vi "Synapse CCD (No Objects).vi"(8 "error in (no error)":errorcluster, 10 "Mono Unique ID":string="Mono1", 11 "Unique ID":string="CCD1") -> (0 "error out":errorcluster, 3 "Synapse CCD out":T1={"JYCCDLib.IJYCCDReqd"=refnum, "JYMONOLib.IJYMonoReqd"=refnum, "Integration time"=0.01, "ADC"=0, "GAIN"=0, "areas :"=[[1, 1, 1, 1024, 256, 1, 256]], "Most Recent Data Object"=refnum, "Mono Properties"={"Grating"=0, "Center Wavelength"=0.0, "Entrance Slit"=0.0, "Exit Slit"=0.0}, "Coverage"={"Max"=0.0, "Min"=0.0}, "Multi-Acquisitions"={"Dark Subtract?"=FALSE, "Averaging?"=FALSE, "Cosmic Ray Removal?"=FALSE, "# to Average"=0, "Time Between Acq."=0, "Acquisitions Control Array"=[TRUE], "Raw Data"=[], "Processed Data"=[], "Array of Wavelengths"=[]}, "Channel Names"=["Wavelength", "Signal"], "Channel Units"=["nm", "counts"]} {"ADC" items=["   20 kHz", "1 MHz", "1 MHz Ultra"]; "GAIN" items=["High Light", "Best Dynamic", "High Sensitivity"]; "Mono Properties"."Grating" items=["1200 lines/mm - 500 nm Blaze", "1200 lines/mm - 750 nm Blaze", "600 lines/mm - 1000 nm Blaze"]})   [LabVIEW 2015]
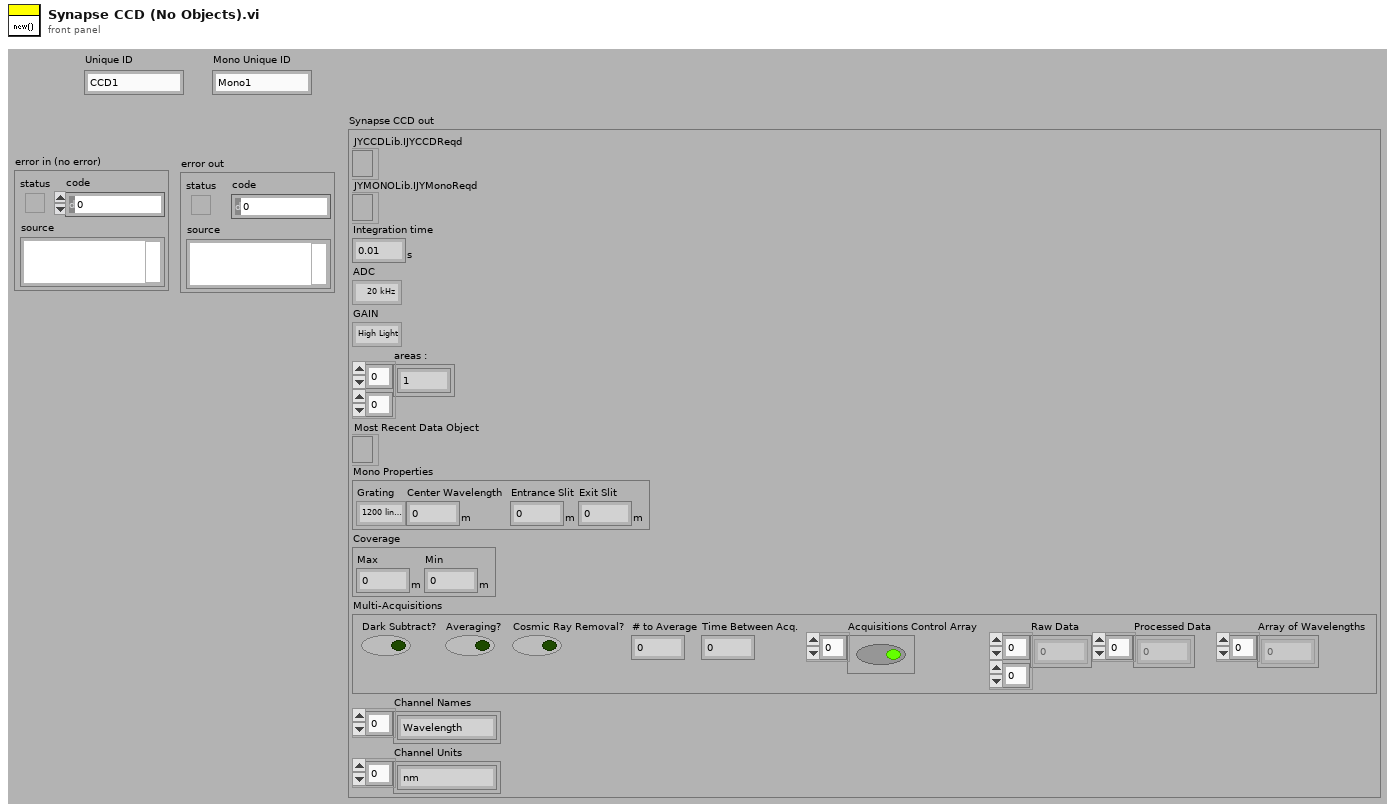
[diagram p1: front panel]
types:
  T1 = cluster{"JYCCDLib.IJYCCDReqd":refnum<k7>, "JYMONOLib.IJYMonoReqd":refnum<k7>, "Integration time":dbl[unit], "ADC":u16, "GAIN":u16, "areas :":i32[][], "Most Recent Data Object":refnum<k7>, "Mono Properties":cluster{"Grating":u16, "Center Wavelength":dbl[unit], "Entrance Slit":dbl[unit], "Exit Slit":dbl[unit]}, "Coverage":cluster{"Max":dbl[unit], "Min":dbl[unit]}, "Multi-Acquisitions":cluster{"Dark Subtract?":bool, "Averaging?":bool, "Cosmic Ray Removal?":bool, "# to Average":u32, "Time Between Acq.":u32, "Acquisitions Control Array":bool[], "Raw Data":i32[][], "Processed Data":dbl[], "Array of Wavelengths":dbl[]}, "Channel Names":string[], "Channel Units":string[]}
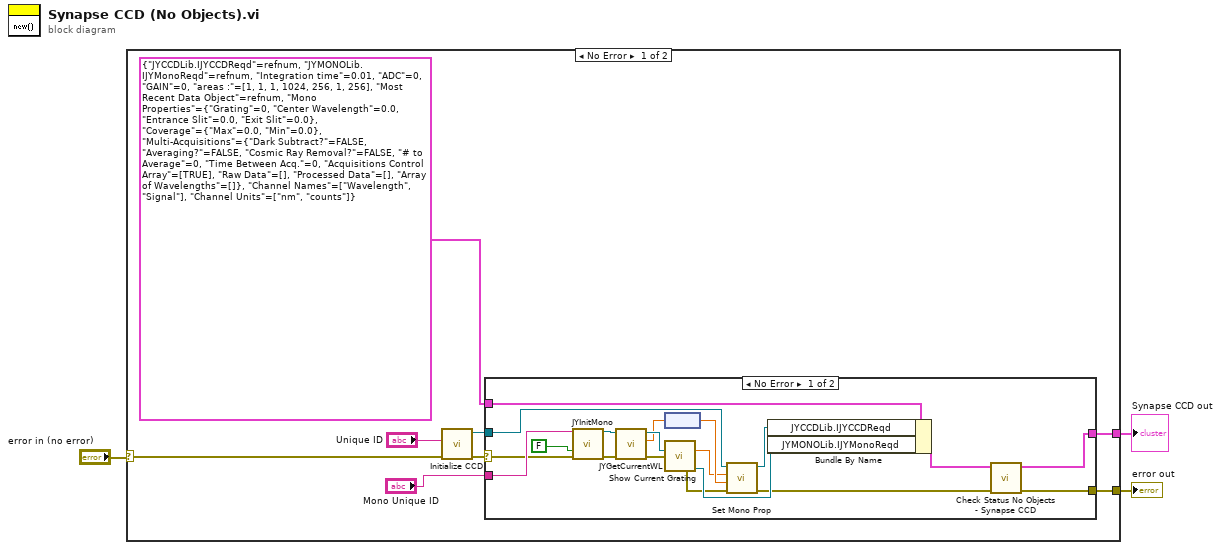
[diagram p0: block diagram]
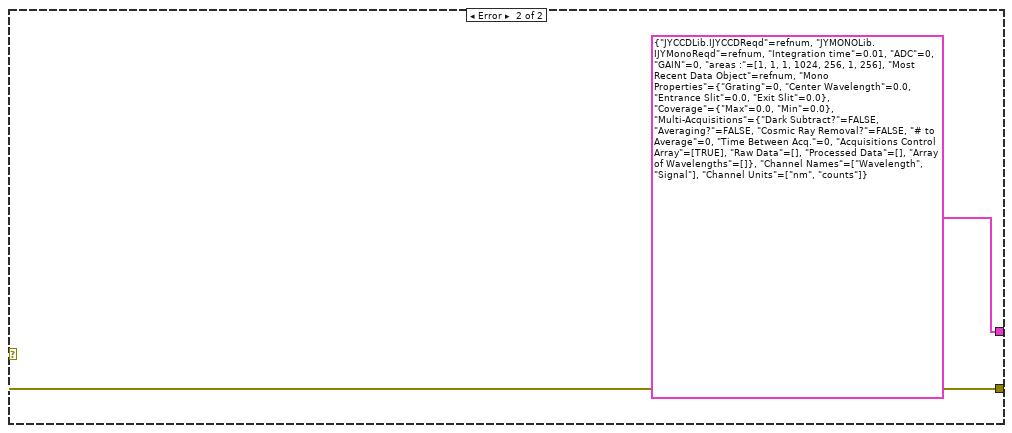
[diagram p3: hidden frame]
diagram:
  n1 = case shown="No Error" "error in (no error)" {
    selector: "error in (no error)" -> [w8 w34]
    tunnel: [w11 T1 {"JYCCDLib.IJYCCDReqd"=refnum, "JYMONOLib.IJYMonoReqd"=refnum, "Integration time"=0.01, "ADC"=0, "GAIN"=0, "areas :"=[[1, 1, 1, 1024, 256, 1, 256]], "Most Recent Data Object"=refnum, "Mono Properties"={"Grating"=0, "Center Wavelength"=0.0, "Entrance Slit"=0.0, "Exit Slit"=0.0}, "Coverage"={"Max"=0.0, "Min"=0.0}, "Multi-Acquisitions"={"Dark Subtract?"=FALSE, "Averaging?"=FALSE, "Cosmic Ray Removal?"=FALSE, "# to Average"=0, "Time Between Acq."=0, "Acquisitions Control Array"=[TRUE], "Raw Data"=[], "Processed Data"=[], "Array of Wavelengths"=[]}, "Channel Names"=["Wavelength", "Signal"], "Channel Units"=["nm", "counts"]} ("Synapse CCD")] -> w2
    tunnel: [w10 w34] -> w3
    frame No Error {
      n2 = call "Initialize CCD.vi"("error in (no error)"=w8, "Unique id:"="Unique ID") -> ("Error out"=w7:errorcluster, "JYCCDLib.IJYCCDReqd Out"=w9:refnum<k7>)  [unwired: 4 in, 4 out]
      n3 = case shown="No Error" w7 {
        selector: w7 -> [w15 w32]
        tunnel: "Mono Unique ID" -> [w30 _]
        tunnel: [w28 w31] -> w11
        tunnel: [w27 w32] -> w10
        tunnel: w9 -> [w17 _]
        tunnel: T1 {"JYCCDLib.IJYCCDReqd"=refnum, "JYMONOLib.IJYMonoReqd"=refnum, "Integration time"=0.01, "ADC"=0, "GAIN"=0, "areas :"=[[1, 1, 1, 1024, 256, 1, 256]], "Most Recent Data Object"=refnum, "Mono Properties"={"Grating"=0, "Center Wavelength"=0.0, "Entrance Slit"=0.0, "Exit Slit"=0.0}, "Coverage"={"Max"=0.0, "Min"=0.0}, "Multi-Acquisitions"={"Dark Subtract?"=FALSE, "Averaging?"=FALSE, "Cosmic Ray Removal?"=FALSE, "# to Average"=0, "Time Between Acq."=0, "Acquisitions Control Array"=[TRUE], "Raw Data"=[], "Processed Data"=[], "Array of Wavelengths"=[]}, "Channel Names"=["Wavelength", "Signal"], "Channel Units"=["nm", "counts"]} ("Synapse CCD") -> [w12 w31]
        frame No Error {
          n4 = call "JYInitMono.vi"("Unique ID"=w30, "Force Init"=FALSE, "error in (no error)"=w15) -> ("Mono RefNum out"=w24:refnum<k7>, "error out"=w26:errorcluster)  [unwired: 8 in, 3 out]
          n5 = call "JYGetCurrentWL.vi"("error in (no error)"=w26, "JYMONOLib.IJYMonoReqd In"=w24) -> ("error out"=w23:errorcluster, "Current WL"=w21:dbl, "JYMONOLib.IJYMonoReqd Out"=w22:refnum<k7>)  [unwired: 6 in, 1 out]
          n6 = node(w21) -> (w20:dbl[unit])
          n7 = call "Show Current Grating.vi"("JYMONOLib.IJYMonoReqd  in"=w22, "error in (no error)"=w23) -> ("Current Grating"=w19:dbl, "error out"=w16:errorcluster, "JYMONOLib.IJYMonoReqd Out"=w18:refnum<k7>)  [unwired: 5 in, 6 out]
          n8 = call "Set Mono Prop.vi"("error in (no error)"=w16, "Current Wavelength"=w20, "Current Grating"=w19, "IJYCCDReqd In"=w17) -> ("error out"=w13:errorcluster, "IJYCCDReqd out"=w25:refnum<k7>)  [unwired: 6 in]
          n9 = Bundle By Name(cluster=w12, "JYCCDLib.IJYCCDReqd"=w25, "JYMONOLib.IJYMonoReqd"=w18) -> (w29:T1)
          n10 = call "Check Status No Objects - Synapse CCD.vi"("error in (no error)"=w13, "Synapse CCD in"=w29) -> ("error out"=w27:errorcluster, "Synapse CCD out"=w28:T1)  [unwired: 6 in, 2 out]
        }
        frame Error {
          # "If CCD doesn't initialize\nproperly, don't do any\nof the mono stuff either."
        }
      }
    }
    frame Error {
    }
  }
  "error out" <- w3
  "Synapse CCD out" <- w2
